vi "Display RT Test.vi"() -> ()   [LabVIEW 2019]
uses:
  Display/Public/Controls/Size.ctl
  Display/Public/Controls/RGB Gains.ctl
  Pixel/Pixel.lvclass
  C:/Users/goo13/Documents/GIT Local/myRIO-Neopixel/Source/RT/Display Element/Display Element.lvclass
  Display Element/Public/Controls/Vector.ctl
  <vilib>/numeric/Random Number (Range) U64.vi
  <vilib>/numeric/Random Number (Range) I64.vi
  <vilib>/numeric/sub_Random U32.vi
  <vilib>/FPGAPlugInAG/myRIO-1900/niLvFpga_Open_myRIO-1900.vi
  <vilib>/rvi/interface/common/dynamic/niFpgaDynamicAddResources.vi
  <vilib>/Utility/error.llb/Error Cluster From Error Code.vi
  <vilib>/rvi/errors/niLvFpgaAdjustHostInterfaceError.vi
  <vilib>/FPGAPlugInAG/Dynamic/niLvFpga_Close_Dynamic.vi
  <vilib>/rvi/interface/nirviOpenFPGA/nirviOpenFPGA.xnode
  FPGA Bitfiles/myrio-neopixel_FPGATarget_TestNeopixel_-8uHP6HNTAw.lvbitx
  <vilib>/rvi/interface/nirviMethod/nirviMethod.xnode
  <vilib>/rvi/interface/nirviReadWriteControl/nirviReadWriteControl.xnode
  <vilib>/rvi/interface/nirviCloseFPGA/nirviCloseFPGA.xnode
  Display/Display.lvclass
  NiFpgaLv.dll
  <vilib>/rvi/interface/Simulation/niFpgaSimulationCallBeginRW.vi
  <vilib>/FPGAPlugInAG/Dynamic/niLvFpga_WriteFifo_Dynamic.vi
  <vilib>/rvi/errors/niLvFpgaMergeErrorWithErrorCode.vi
  Display Element/Display Element.lvclass
panel:
  in  "Intensity":sgl(slide)=0.5 scale=0.0..1.0
  in  "FPS":u32(slide)=40 scale=0.0..400.0
  in  "stop":bool
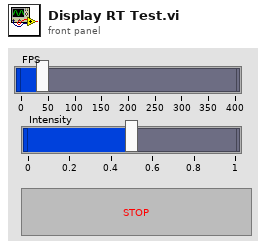
[diagram p1: front panel]
types:
  T1 = typedef "Display.lvclass/Size.ctl" = cluster{"Width":i32, "Height":i32}
  T2 = typedef "Display.lvclass/RGB Gains.ctl" = cluster{"Red":sgl, "Green":sgl, "Blue":sgl}
  T3 = typedef "Display Element.lvclass/Vector.ctl" = cluster{"X":i32, "Y":i32}
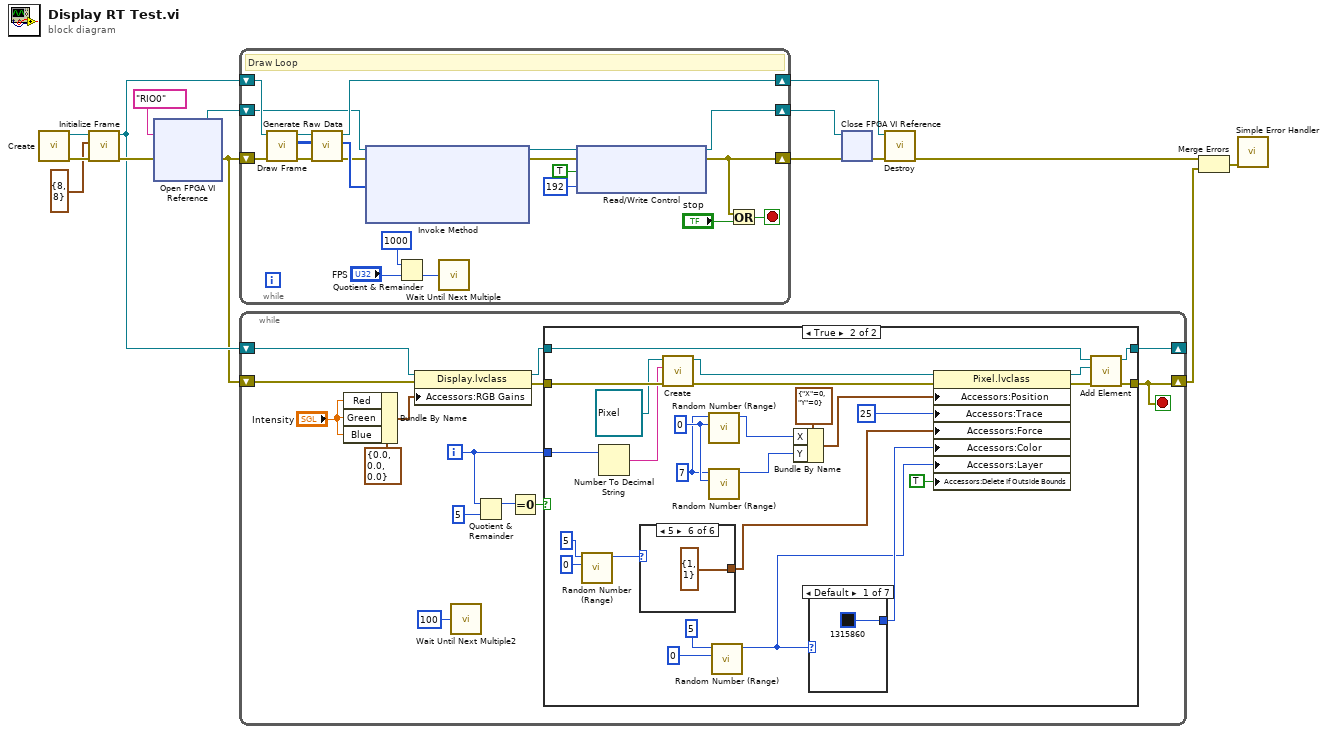
[diagram p0: block diagram]
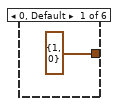
[diagram p3: hidden frame]
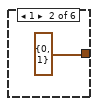
[diagram p4: hidden frame]
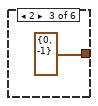
[diagram p5: hidden frame]
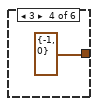
[diagram p6: hidden frame]
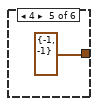
[diagram p7: hidden frame]
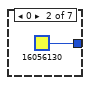
[diagram p8: hidden frame]
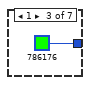
[diagram p9: hidden frame]
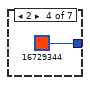
[diagram p10: hidden frame]
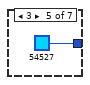
[diagram p11: hidden frame]
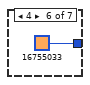
[diagram p12: hidden frame]
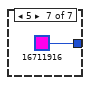
[diagram p13: hidden frame]
diagram:
  n1 = call "Create.vi"() -> ("Error Out"=w10:errorcluster, "Screen Out"=w11:refnum<class "Display.lvclass">)  [unwired: 10 in]
  n2 = call "Initialize Frame.vi"("Error In"=w10, "Size"=T1 {"Width"=8, "Height"=8}, "Display In"=w11) -> ("Error Out"=w8:errorcluster, "Display Out"=w7:refnum<class "Display.lvclass">)  [unwired: 7 in]
  n3 = xnode "Open FPGA VI Reference"("error in"=w8, "resource name"=tag "RIO0") -> ("FPGA VI Reference Out"=w14:refnum<k20>, "error out"=w4:errorcluster)
  n4 = while {
    shift-right: [w35] -> w13
    shift-left: w14 -> [w23]
    shift-right: [w17] -> w12
    shift-left: w4 -> [w31]
    shift-right: [w26] -> w6
    shift-left: w7 -> [w30]
    stop <- w18 stop-if-true
    # "Draw Loop"
    n5 = call "Draw Frame.vi"("Error In"=w31, "Display In"=w30) -> ("Error Out"=w29:errorcluster, "Frame"=w27:u32[][], "Display Out"=w28:refnum<class "Display.lvclass">)  [unwired: 7 in]
    n6 = call "Generate Raw Data.vi"("Error In"=w29, "Matrix"=w27, "Display In"=w28) -> ("Error Out"=w19:errorcluster, "Raw Data"=w20:u8[], "Display Out"=w26:refnum<class "Display.lvclass">)  [unwired: 6 in]
    n7 = xnode "Invoke Method"("FPGA VI Reference In"=w23, "error in"=w19, "Data"=w20) -> ("FPGA VI Reference Out"=w22:refnum<k20>, "error out"=w21:errorcluster)  [unwired: 1 in, 1 out]
    n8 = Quotient & Remainder(x=u32 1000 ("y"), y="FPS") -> (floor(x/y)=w32:u32)  [unwired: 1 out]
    n9 = call "Wait Until Next Multiple"("Count(mSec)"=w32) -> ()  [unwired: 1 out]
    n10 = xnode "Read/Write Control"("FPGA VI Reference In"=w22, "error in"=w21, "Update"=TRUE, "Number Of Elements"=192) -> ("FPGA VI Reference Out"=w35:refnum<k20>, "error out"=w17:errorcluster)
    n11 = Or(x=w17, y="stop") -> (x .or. y?=w18:bool)
  }
  n12 = while {
    shift-right: [w41] -> _
    shift-left: w7 -> [w49]
    shift-right: [w42] -> w2
    shift-left: w4 -> [w46]
    i -> [w40]
    stop <- w42 stop-if-true
    n13 = Bundle By Name(cluster=T2 {"Red"=0.0, "Green"=0.0, "Blue"=0.0} ("RGB Gains"), "Red"="Intensity", "Green"="Intensity", "Blue"="Intensity") -> (w47:T2)
    n14 = property class="Display.lvclass"(reference=w49, error in=w46, "Accessors:RGB Gains"=w47) -> (reference out=w43:refnum<class "Display.lvclass">, error out=w44:errorcluster)
    n15 = call "Wait Until Next Multiple2"("Count(mSec)"=u32 100) -> ()  [unwired: 1 out]
    n16 = Quotient & Remainder(x=w40, y=5) -> (x-y*floor(x/y)=w37:i32)  [unwired: 1 out]
    n17 = Equal To 0?(x=w37) -> (x = 0?=w36:bool)
    n18 = case shown="True" w36 {
      tunnel: w44 -> [w50 w78]
      tunnel: w40 -> [_ w76]
      tunnel: w43 -> [w51 w74]
      tunnel: [w51 w73] -> w41
      tunnel: [w50 w72] -> w42
      frame False {
      }
      frame True {
        w57 = u64 7 ("upper bound (100)")
        w62 = u64 0 ("lower bound (0)")
        n19 = call-poly <vilib>:"Random Number (Range).vi"("lower bound (0)"=u64 0, "upper bound (100)"=u64 5) -> ("number"=w54:u64)  [unwired: 9 in]
        n20 = Number To Decimal String(number=w76) -> (decimal integer string=w75:string)  [unwired: 1 in]
        n21 = case shown="5" w54 {
          tunnel: [T3 {"X"=1, "Y"=0} ("Position") T3 {"X"=0, "Y"=1} ("Position") T3 {"X"=0, "Y"=-1} ("Position") T3 {"X"=-1, "Y"=0} ("Position") T3 {"X"=-1, "Y"=-1} ("Position") T3 {"X"=1, "Y"=1} ("Position")] -> w53
          frame 0, Default {
          }
          frame 1 {
          }
          frame 2 {
          }
          frame 3 {
          }
          frame 4 {
          }
          frame 5 {
          }
        }
        n22 = call-dynamic "Create.vi"("Error In"=w78, "Tag"=w75, "Pixel In"=refnum<class "Pixel.lvclass"> refnum) -> ("Error Out"=w70:errorcluster, "Pixel Out"=w71:refnum<class "Pixel.lvclass">)  [unwired: 7 in]
        n23 = call-poly <vilib>:"Random Number (Range).vi"("lower bound (0)"=w62, "upper bound (100)"=w57) -> ("number"=w66:u64)  [unwired: 9 in]
        n24 = call-poly <vilib>:"Random Number (Range).vi"("lower bound (0)"=w62, "upper bound (100)"=w57) -> ("number"=w65:u64)  [unwired: 9 in]
        n25 = call-poly <vilib>:"Random Number (Range).vi"("lower bound (-100)"=i64 0, "upper bound (100)"=i64 5) -> ("number"=w58:i64)  [unwired: 9 in]
        n26 = Bundle By Name(cluster=T3 {"X"=0, "Y"=0} ("Position"), "X"=w66, "Y"=w65) -> (w64:T3)
        n27 = case shown="Default" w58 {
          tunnel: [u32 1315860 ("Color") u32 16056130 ("Color") u32 786176 ("Color") u32 16729344 ("Color") u32 54527 ("Color") u32 16755033 ("Color") u32 16711916 ("Color")] -> w59
          frame Default {
          }
          frame 0 {
          }
          frame 1 {
          }
          frame 2 {
          }
          frame 3 {
          }
          frame 4 {
          }
          frame 5 {
          }
        }
        n28 = property class="Pixel.lvclass"(reference=w71, error in=w70, "Accessors:Position"=w64, "Accessors:Trace"=25 ("Trace"), "Accessors:Force"=w53, "Accessors:Color"=w59, "Accessors:Layer"=w58, "Accessors:Delete If Outside Bounds"=TRUE ("Delete If Outside Bounds")) -> (reference out=w69:refnum<class "Pixel.lvclass">, error out=w68:errorcluster)
        n29 = call "Add Element.vi"("Error In"=w68, "New Element"=w69, "Display In"=w74) -> ("Error Out"=w72:errorcluster, "Display Out"=w73:refnum<class "Display.lvclass">)  [unwired: 7 in]
      }
    }
  }
  n30 = xnode "Close FPGA VI Reference"("FPGA VI Reference In"=w13, "error in"=w12) -> ("error out"=w5:errorcluster)
  n31 = call "Destroy.vi"("Error In"=w5, "Display In"=w6) -> ("Error Out"=w3:errorcluster)  [unwired: 9 in]
  n32 = Merge Errors(w3, w2) -> (w1:errorcluster)
  n33 = call <vilib>:"Simple Error Handler.vi"("error in (no error)"=w1) -> ()  [unwired: 4 in, 5 out]
